vi "Build Spec-Type.vi"(8 "error in (no error)":errorcluster, 10 "Type":string="Packed Library", 11 "Path to project":path) -> (0 "error out":errorcluster, 2 "Generated files":path[](array[path]))   [LabVIEW 2022 SP3]
uses:
  <vilib>/AppBuilder/AB_API_Simple/Build (path).vi
  <vilib>/AppBuilder/AB_API_Simple/NI_App_Builder_API.lvlib
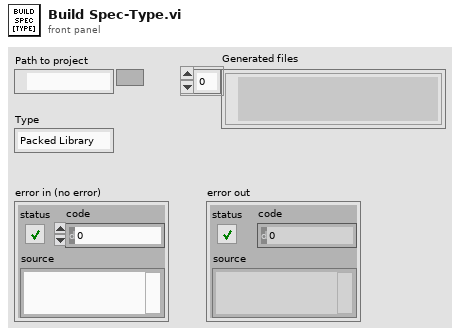
[diagram p1: front panel]
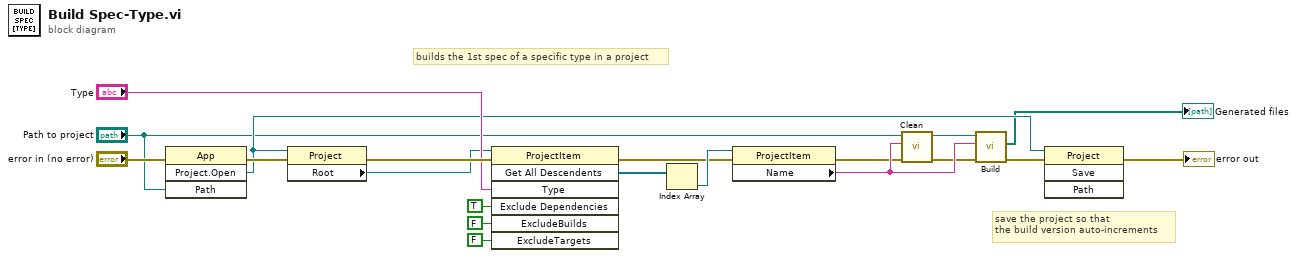
[diagram p0: block diagram]
diagram:
  # "save the project so that\nthe build version auto-increments"
  # "builds the 1st spec of a specific type in a project"
  n1 = invoke class="App" method="Project.Open"(error in="error in (no error)", "Path"="Path to project") -> (error out=w9:errorcluster, "Project:Open"=w7:refnum<vi>)  [unwired: 2 in, 2 out]
  n2 = property class="Project"(reference=w7, error in=w9) -> (error out=w15:errorcluster, "Root"=w10:refnum<vi>)  [unwired: 1 out]
  n3 = invoke class="ProjectItem" method="Get All Descendents"(reference=w10, error in=w15, "Type"="Type", "Exclude Dependencies"=TRUE ("ExcludeDependencies"), "ExcludeBuilds"=FALSE, "ExcludeTargets"=FALSE) -> (error out=w16:errorcluster, "All Descendents"=w17:refnum<vi>[])  [unwired: 1 in, 5 out]
  n4 = Index Array(array=w17) -> (element=w18:refnum<vi>)  [unwired: 1 in]
  n5 = property class="ProjectItem"(reference=w18, error in=w16) -> (error out=w3:errorcluster, "Name"=w4:string)  [unwired: 1 out]
  n6 = call <vilib>:"Clean.vi"("error in (no error)"=w3, "Name of build specification (if empty: clean all)"=w4, "Path to project"="Path to project") -> ("error out"=w2:errorcluster)  [unwired: 8 in]
  n7 = call-poly <vilib>:"Build.vi"("error in (no error)"=w2, "Name of build specification (if empty: build all)"=w4, "Path to project"="Path to project") -> ("error out"=w8:errorcluster, "Generated files"=→"Generated files":path[])  [unwired: 7 in]
  n8 = invoke class="Project" method="Save"(reference=w7, error in=w8) -> (error out=→"error out":errorcluster)  [unwired: 2 in, 3 out]
